vi "LoadPanel.vi"(0 "VI in":refnum<vi>, 5 "Item Name":string, 11 "error in":errorcluster) -> (4 "VI out":refnum<vi>, 15 "error out":errorcluster)   [LabVIEW 2016, in "DronaTest.lvlib"]
uses:
  DronaTest.lvlib
  APIs/Stimulus/ControlValue/ValueSignalByPathString.vi
  APIs/Stimulus/ControlValue/Controls/Listbox/SetValueByItemName.vi
  Drona.lvlib
  APIs/Stimulus/ControlValue/Controls/Listbox/StimulusListbox.lvlib
  APIs/Stimulus/ControlValue/ControlValue.lvlib
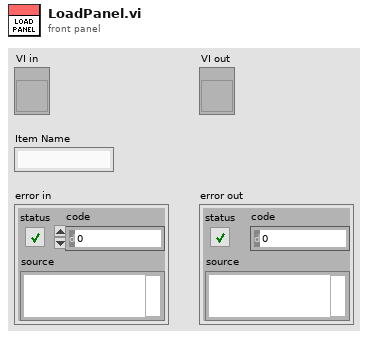
[diagram p1: front panel]
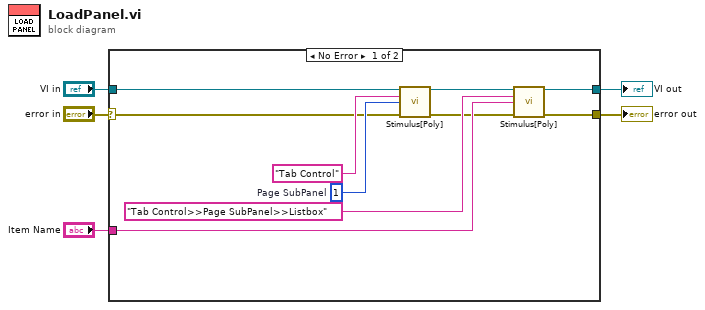
[diagram p0: block diagram]
diagram:
  n1 = case shown="No Error" "error in" {
    selector: "error in" -> [w6 w16]
    tunnel: [w15 w17] -> w5
    tunnel: [w14 w16] -> w4
    tunnel: "VI in" -> [w13 w17]
    tunnel: "Item Name" -> [w10 _]
    frame No Error {
      w11 = 1  # Page SubPanel
      n2 = call-poly "Stimulus[Poly].vi"("VI Reference In"=w13, "Control Path"="Tab Control", "Value (Signaling)"=w11, "error in"=w6) -> ("VI Reference Out"=w7:refnum<vi>, "error out"=w8:errorcluster)  [unwired: 10 in]
      n3 = call-poly "Stimulus[Poly].vi"("VI Reference In"=w7, "Control Path"="Tab Control>>Page SubPanel>>Listbox", "Item Name"=w10, "Error In"=w8) -> ("VI Reference Out"=w15:refnum<vi>, "Error Out"=w14:errorcluster)  [unwired: 10 in]
    }
    frame Error {
    }
  }
  "VI out" <- w5
  "error out" <- w4
